vi "Async-Message with Queue.vi"() -> ()   [LabVIEW 2020, in "TCPRouter ClientAPI Examples.lvlib"]
uses:
  _addons/TCP-Router/ClientAPI/Def-TCP-Router Async-Resp Data.ctl
  b3b63605-1016-4be4-a788-12e3256b011c.vi
  TCPRouter ClientAPI Examples.lvlib
  _addons/TCP-Router/ClientAPI/TcpRouter-Client.lvclass
panel:
  out "element":T1[](array[typedef])
  out "# elements in queue":i32
  out "current time":timestamp
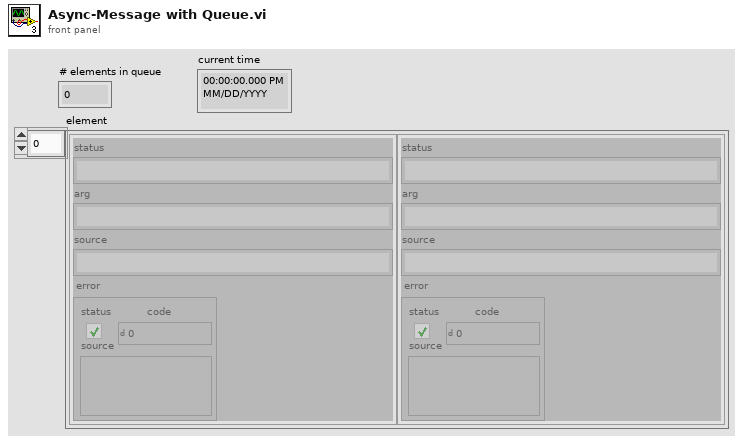
[diagram p1: front panel]
types:
  T1 = typedef "CSM-TCP-Router.lvlib/TcpRouter-Client.lvclass/Def-TCP-Router Async-Resp Data.ctl" = cluster{"status":string, "arg":string, "source":string, "error":errorcluster}
  T2 = cluster{"IP Address":string, "Port":u16, "ConnectTMO":i32}
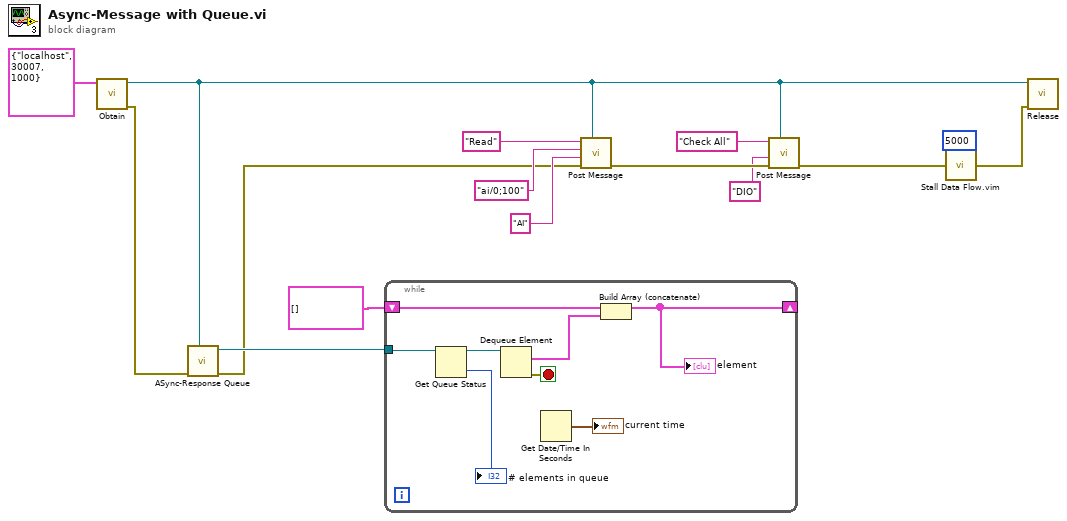
[diagram p0: block diagram]
diagram:
  n1 = call "Obtain.vi"("Connection"=T2 {"IP Address"="localhost", "Port"=30007, "ConnectTMO"=1000}) -> ("error out"=w11:errorcluster, "TcpRouter-Client out"=w2:refnum<class "TcpRouter-Client.lvclass">)  [unwired: 9 in]
  n2 = call "ASync-Response Queue.vi"("TcpRouter-Client in"=w2, "error in (no error)"=w11) -> ("error out"=w3:errorcluster, "ASync-Resp Queue"=w12:refnum<queue>)  [unwired: 8 in]
  n3 = while {
    tunnel: w12 -> [w23]
    shift-right: [w17] -> _
    shift-left: T1[] [] ("element") -> [w18]
    stop <- w22 stop-if-true
    n4 = Get Queue Status(queue=w23) -> (queue out=w20:refnum<queue>, # elements in queue=→"# elements in queue":i32)  [unwired: 2 in, 6 out]
    n5 = Dequeue Element(queue=w20) -> (element=w16:T1, error out=w22:errorcluster)  [unwired: 2 in, 2 out]
    n6 = Get Date/Time In Seconds() -> (seconds since 1Jan1904=→"current time":timestamp)
    n7 = Build Array (concatenate)(w18, w16) -> (w17:T1[])
    "element" <- w17
  }
  n8 = call "Post Message.vi"("TcpRouter-Client in"=w2, "error in (no error)"=w3, "Target Module"="AI", "Arguments (\"\")"="ai/0;100" ("State"), "State"="Read") -> ("error out"=w7:errorcluster)  [unwired: 6 in]
  n9 = call "Post Message.vi"("TcpRouter-Client in"=w2, "error in (no error)"=w7, "Target Module"="DIO", "State"="Check All") -> ("error out"=w4:errorcluster)  [unwired: 7 in]
  n10 = call "Stall Data Flow.vim"("value in"=w4, "milliseconds to wait"=u32 5000) -> ("value out"=w14:errorcluster)  [unwired: 1 out]
  n11 = call "Release.vi"("error in (no error)"=w14, "TcpRouter-Client in"=w2) -> ()  [unwired: 9 in, 1 out]
